vi "Assignment3_1.vi"() -> ()   [LabVIEW 2025]
doc: "This VI Inverts the Input String \nif A ----> a\nif b ----> B"
panel:
  in  "STOP":bool
  in  "Input String":string
  # "Simulating Caps Lock event in Keyboard."
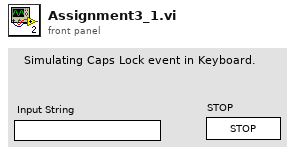
[diagram p1: front panel]
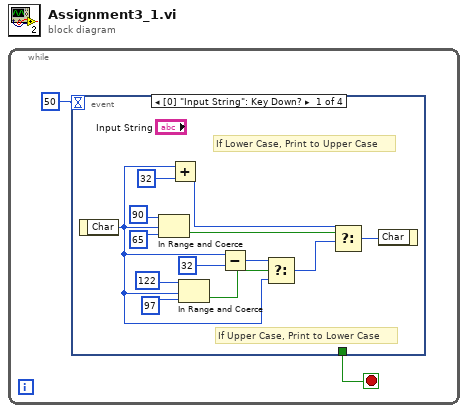
[diagram p0: block diagram]
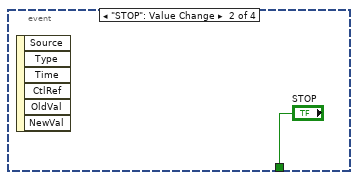
[diagram p2: hidden frame]
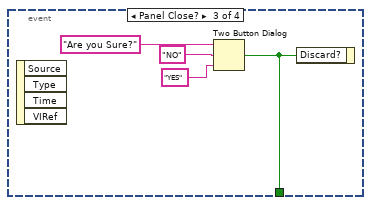
[diagram p3: hidden frame]
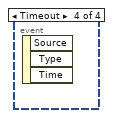
[diagram p4: hidden frame]
diagram:
  n1 = while {
    stop <- w2 stop-if-true
    n2 = event shown="[0] \"Input String\": Key Down?" {
      selector: _ -> [_ _ _ _]
      dyn-events: _ -> [_ _ _ _]
      timeout: 50 -> [_ _ _ _]
      tunnel: [_ "STOP" w17 _] -> w2
      event "Input String": Key Down? {
        # "If Upper Case, Print to Lower Case"
        # "If Lower Case, Print to Upper Case"
        n3 = event-data() -> ("Char"=w4:i16)  [unwired: 1 in]
        n4 = In Range and Coerce(upper limit=i16 90, x=w4, lower limit=i16 65) -> (In Range?=w13:bool)  [unwired: 1 out]
        n5 = Add(x=w4, y=i16 32) -> (x+y=w11:i16)
        n6 = In Range and Coerce(upper limit=i16 122, x=w4, lower limit=i16 97) -> (In Range?=w8:bool)  [unwired: 1 out]
        n7 = Subtract(x=w4, y=i16 32) -> (x-y=w6:i16)
        n8 = Select(t=w6, s=w8, f=w4) -> (s? t:f=w5:i16)
        n9 = Select(t=w11, s=w13, f=w5) -> (s? t:f=w3:i16)
        n10 = event-data("Char"=w3) -> ()  [unwired: 1 in, 1 out]
      }
      event "STOP": Value Change {
        n11 = event-data() -> ()  [unwired: 1 in, 6 out]
      }
      event Panel Close? {
        n12 = event-data() -> ()  [unwired: 1 in, 4 out]
        n13 = Two Button Dialog(message="Are you Sure?", 1:"YES" ("F button name (\"Cancel\")"), 2:"NO" ("T button name (\"OK\")")) -> (T button?=w17:bool)
        n14 = event-data("Discard?"=w17) -> ()  [unwired: 1 in, 1 out]
      }
      event Timeout {
        n15 = event-data() -> ()  [unwired: 1 in, 3 out]
      }
    }
  }
